vi "SubILoss.vi"() -> ()   [LabVIEW 2022 SP3]
uses:
  <vilib>/Utility/file.llb/Read From Spreadsheet File (DBL).vi
  <vilib>/Utility/file.llb/Write To Spreadsheet File (DBL).vi
panel:
  out "Rcv":dbl[](graph)
  out "Xmit":dbl[](graph)
  in  "Boolean":bool
  out "IL":cluster{"all rows":dbl[], dbl[]}(graph)
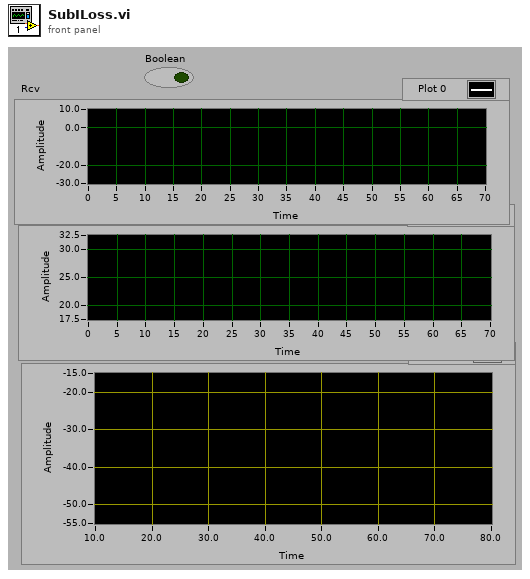
[diagram p1: front panel]
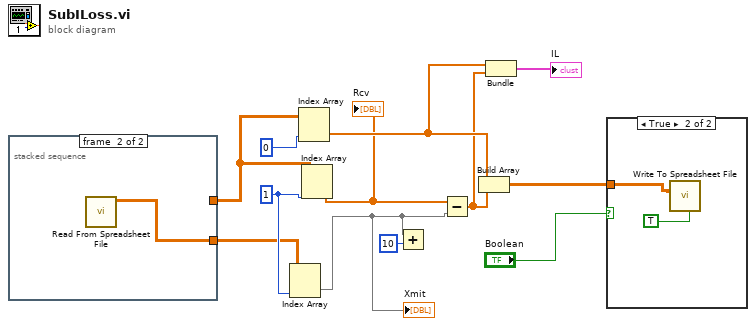
[diagram p0: block diagram]
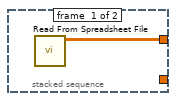
[diagram p3: hidden frame]
diagram:
  w10 = 1
  n1 = stacked-sequence {
    tunnel: [w13 _] -> w12
    tunnel: [_ w14] -> w9
    frame #0 {
      n2 = call-poly <vilib>:"Read From Spreadsheet File.vi"() -> ("all rows"=w13:dbl[][])  [unwired: 4 in, 7 out]
    }
    frame #1 {
      n3 = call-poly <vilib>:"Read From Spreadsheet File.vi"() -> ("all rows"=w14:dbl[][])  [unwired: 4 in, 7 out]
    }
  }
  n4 = Index Array(array=w9, index (col)=w10) -> (element=w1:dbl[])  [unwired: 1 in]
  "Xmit" <- w1
  n5 = Index Array(array=w12, index (col)=0) -> (element=w8:dbl[])  [unwired: 1 in]
  n6 = Index Array(array=w12, index (col)=w10) -> (element=w3:dbl[])  [unwired: 1 in]
  "Rcv" <- w3
  n7 = Add(x=w1, y=10) -> ()  [unwired: 1 out]
  n8 = Subtract(x=w3, y=w1) -> (x-y=w7:dbl[])
  n9 = Build Array(w8, w7) -> (w5:dbl[][])
  n10 = Bundle("all rows"=w8, w7) -> (→"IL":cluster{"all rows":dbl[], dbl[]})  [unwired: 1 out]
  n11 = case shown="True" "Boolean" {
    tunnel: w5 -> [_ w16]
    frame False {
    }
    frame True {
      n12 = call-poly <vilib>:"Write To Spreadsheet File.vi"("transpose? (no:F)"=TRUE, "2D data"=w16) -> ()  [unwired: 4 in, 3 out]
    }
  }
